vi "RT Main.vi"   [LabVIEW 2019]
uses:
  <vilib>/FPGAPlugInAG/myRIO-1900/niLvFpga_Open_myRIO-1900.vi
  <vilib>/rvi/interface/common/dynamic/niFpgaDynamicAddResources.vi
  <vilib>/Utility/error.llb/Error Cluster From Error Code.vi
  <vilib>/rvi/errors/niLvFpgaAdjustHostInterfaceError.vi
  <vilib>/FPGAPlugInAG/Dynamic/niLvFpga_Close_Dynamic.vi
  <vilib>/rvi/interface/nirviOpenFPGA/nirviOpenFPGA.xnode
  FPGA Bitfiles/firstFPGAapplica_FPGATarget_FPGAMain_SzxPrRGxuPY.lvbitx
  FPGA Main.vi
  <vilib>/rvi/interface/nirviReadWriteControl/nirviReadWriteControl.xnode
  <vilib>/rvi/interface/nirviCloseFPGA/nirviCloseFPGA.xnode
  NiFpgaLv.dll
  <vilib>/rvi/interface/Simulation/niFpgaSimulationCallBeginRW.vi
panel:
  # "RT startup VI"
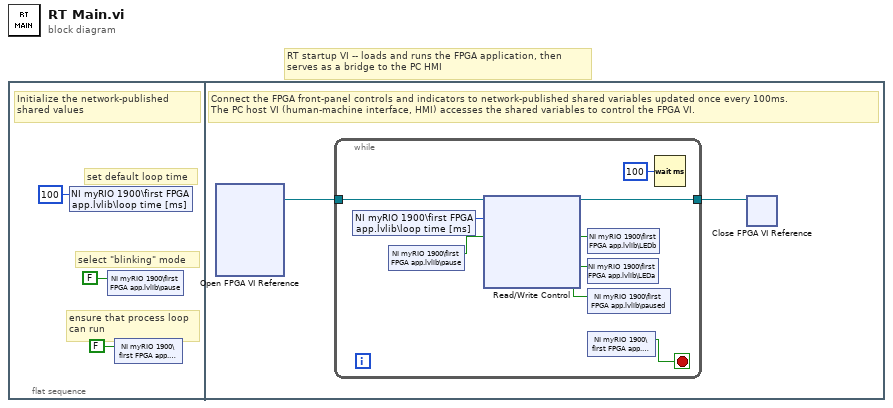
[diagram p0: block diagram]
diagram:
  # "RT startup VI -- loads and runs the FPGA application, then\nserves as a bridge to the PC HMI"
  n1 = flat-sequence {
    frame #0 {
      # "ensure that process loop\ncan run"
      # "select \"blinking\" mode"
      # "set default loop time"
      # "Initialize the network-published\nshared values"
      n2 = shared-variable "NI myRIO 1900\\first FPGA app.lvlib\\loop time [ms]"(u32 100 ("loop time [ms]")) -> ()  [unwired: 1 in, 1 out]
      n3 = shared-variable "NI myRIO 1900\\first FPGA app.lvlib\\pause"(FALSE ("pause")) -> ()  [unwired: 1 in, 1 out]
      n4 = shared-variable "NI myRIO 1900\\first FPGA app.lvlib\\stop"(FALSE ("stop")) -> ()  [unwired: 1 in, 1 out]
    }
    frame #1 {
      # "Connect the FPGA front-panel controls and indicators to network-published shared variables updated once every 100ms.\nThe PC host VI (human-machine interface, HMI) accesses the shared variables to control the FPGA VI."
      n5 = xnode "Open FPGA VI Reference"() -> ("FPGA VI Reference Out"=w5:refnum<k20>)  [unwired: 2 in, 1 out]
      n6 = while {
        tunnel: w5 -> [w14]
        tunnel: [w13] -> w4
        stop <- w7 stop-if-true
        n7 = shared-variable "NI myRIO 1900\\first FPGA app.lvlib\\loop time [ms]"() -> (w11:u32)  [unwired: 1 in, 1 out]
        n8 = shared-variable "NI myRIO 1900\\first FPGA app.lvlib\\pause"() -> (w6:bool)  [unwired: 1 in, 1 out]
        n9 = xnode "Read/Write Control"("FPGA VI Reference In"=w14, "loop time [ms]"=w11, "pause"=w6) -> ("FPGA VI Reference Out"=w13:refnum<k20>, "LEDa"=w10:bool, "LEDb"=w9:bool, "paused"=w8:bool)  [unwired: 1 in, 1 out]
        n10 = shared-variable "NI myRIO 1900\\first FPGA app.lvlib\\LEDb"(w10) -> ()  [unwired: 1 in, 1 out]
        n11 = shared-variable "NI myRIO 1900\\first FPGA app.lvlib\\LEDa"(w9) -> ()  [unwired: 1 in, 1 out]
        n12 = shared-variable "NI myRIO 1900\\first FPGA app.lvlib\\paused"(w8) -> ()  [unwired: 1 in, 1 out]
        n13 = shared-variable "NI myRIO 1900\\first FPGA app.lvlib\\stop"() -> (w7:bool)  [unwired: 1 in, 1 out]
        n14 = Wait (ms)(milliseconds to wait=u32 100) -> ()  [unwired: 1 out]
      }
      n15 = xnode "Close FPGA VI Reference"("FPGA VI Reference In"=w4) -> ()  [unwired: 1 in, 1 out]
    }
  }
